vi "LFA_Initialize.vi"(8 "error in (no error)":errorcluster, 10 "Is Visible?":bool=TRUE, 11 "LightField Automation in":refnum<class "LightField Automation.lvclass">) -> (0 "error out":errorcluster, 3 "LightField Automation out":refnum<class "LightField Automation.lvclass">)   [LabVIEW 2013, in "LightField Automation.lvclass"]
uses:
  LightField Automation.lvclass
  C:/Program Files/Princeton Instruments/LightField/AddInViews/PrincetonInstruments.LightFieldViewV3.dll
  Program Files/Princeton Instruments/LightField/AddInViews/PrincetonInstruments.LightFieldViewV3.dll
  C:/Program Files/Princeton Instruments/LightField/PrincetonInstruments.LightField.AutomationV3.dll
  Program Files/Princeton Instruments/LightField/PrincetonInstruments.LightField.AutomationV3.dll
  LightField Automation.lvclass/LightField Automation.ctl
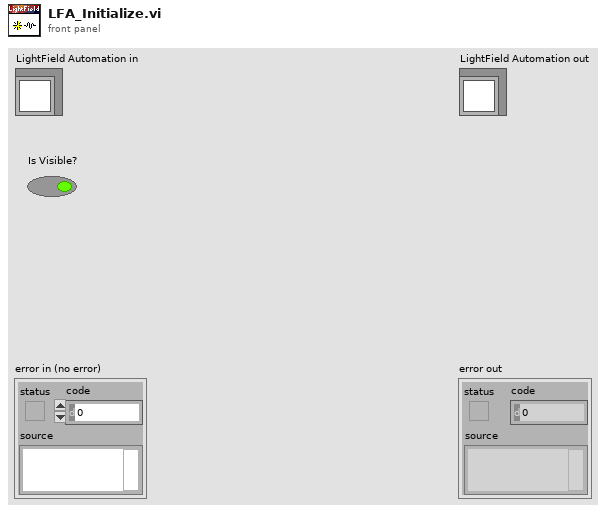
[diagram p1: front panel]
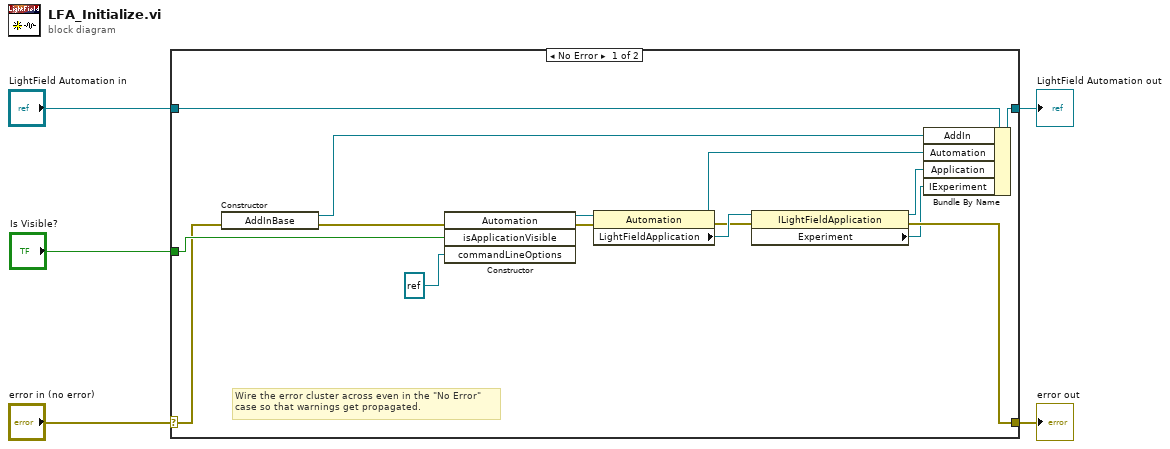
[diagram p0: block diagram]
diagram:
  n1 = case shown="No Error" "error in (no error)" {
    selector: "error in (no error)" -> [w8 w22]
    tunnel: [w18 w22] -> w4
    tunnel: [w16 w21] -> w2
    tunnel: "LightField Automation in" -> [w17 w21]
    tunnel: "Is Visible?" -> [w9 _]
    frame No Error {
      # "Wire the error cluster across even in the \"No Error\"\ncase so that warnings get propagated."
      n2 = constructor class="AddInBase"(error in=w8) -> (reference out=w6:refnum<k24>, error out=w7:errorcluster)  [unwired: 2 in, 1 out]
      n3 = constructor class="Automation"(error in=w7, "isApplicationVisible"=w9, "commandLineOptions"=refnum<k24> refnum) -> (reference out=w12:refnum<k24>, error out=w19:errorcluster)  [unwired: 2 in, 3 out]
      n4 = property class="Automation"(reference=w12, error in=w19) -> (reference out=w13:refnum<k24>, error out=w10:errorcluster, "LightFieldApplication"=w11:refnum<k24>)
      n5 = property class="ILightFieldApplication"(reference=w11, error in=w10) -> (reference out=w14:refnum<k24>, error out=w18:errorcluster, "Experiment"=w15:refnum<k24>)
      n6 = Bundle By Name(cluster=w17, "AddIn"=w6, "Automation"=w13, "Application"=w14, "IExperiment"=w15) -> (w16:refnum<class "LightField Automation.lvclass">)
    }
    frame Error {
    }
  }
  "error out" <- w4
  "LightField Automation out" <- w2
